vi "DQMH Controls Panel.vi"() -> ()   [LabVIEW 2019, in "Panther Dashboard.lvlib"]
uses:
  Panther Dashboard.lvlib
  Controls/Add.ctl
  Controls/Trash.ctl
  Controls/Convert.ctl
  Controls/rename.ctl
  Controls/Unit Testing.ctl
  Controls/Template.ctl
  Controls/Validate.ctl
  Controls/tester.ctl
  Controls/Antidoc.ctl
  Controls/Info.ctl
  Controls/Theme.ctl
  Controls/Open Document.ctl
  DQMH Tools Menu--enum.ctl
panel:
  in  "Open Documentation":T1 caption="Open\nDocumentation"
  in  "Theme":T2
  in  "About":T3
  in  "Add Event":T4 caption="Add\nEvent"
  in  "Remove Event":T5 caption="Remove\nEvent"
  in  "Convert Event":T6 caption="Convert\nEvent"
  in  "Rename Event":T7 caption="Rename\nEvent"
  in  "Add Module":T4 caption="Add\nModule"
  in  "Rename Module":T7 caption="Rename\nModule"
  in  "Validate Module":T8 caption="Validate\nModule"
  in  "Create Module Template":T9 caption="Create\nTemplate"
  in  "Add Unit Test":T10 caption="Add \nUnit Test"
  in  "Create RT Tester":T11 caption="Create RT\nTester"
  in  "Generate Antidoc":T12 caption="Generate\nAntidoc"
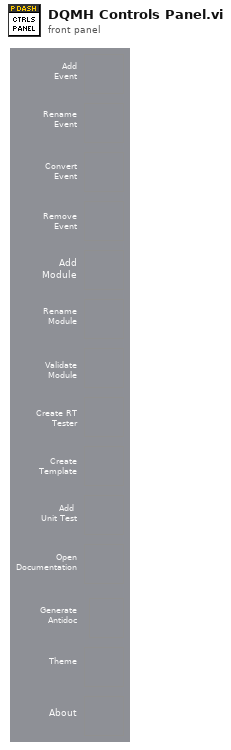
[diagram p1: front panel]
types:
  T1 = typedef "Open Document.ctl" = bool
  T2 = typedef "Theme.ctl" = bool
  T3 = typedef "Info.ctl" = bool
  T4 = typedef "Add.ctl" = bool
  T5 = typedef "Trash.ctl" = bool
  T6 = typedef "Convert.ctl" = bool
  T7 = typedef "rename.ctl" = bool
  T8 = typedef "Validate.ctl" = bool
  T9 = typedef "Template.ctl" = bool
  T10 = typedef "Unit Testing.ctl" = bool
  T11 = typedef "tester.ctl" = bool
  T12 = typedef "Antidoc.ctl" = bool
  T13 = typedef "Panther Dashboard.lvlib/Broadcast Events--cluster.ctl" = cluster{"Module Did Init":refnum<user-event>, "Status Updated":refnum<user-event>, "Error Reported":refnum<user-event>, "Module Did Stop":refnum<user-event>, "Update Module Execution Status":refnum<user-event>, "References Updated":refnum<user-event>, "Projects Updated":refnum<user-event>, "Targets Updated":refnum<user-event>, "Progress updated":refnum<user-event>, "Scale Updated":refnum<user-event>, "Connector Pane Updated":refnum<user-event>, "Documentation Updated":refnum<user-event>, "Module Type Updated":refnum<user-event>}
  T14 = typedef "Panther Dashboard.lvlib/DQMH Tools Menu--enum.ctl" = enum16{"Create New DQMH Event", "Remove DQMH Event", "Convert DQMH Event", "Rename DQMH Event", "Add New DQMH Module", "Create RT Tester", "Rename DQMH Module", "Validate DQMH Module", "Create DQMH Module Template", "New DQMH  Unit Test"}
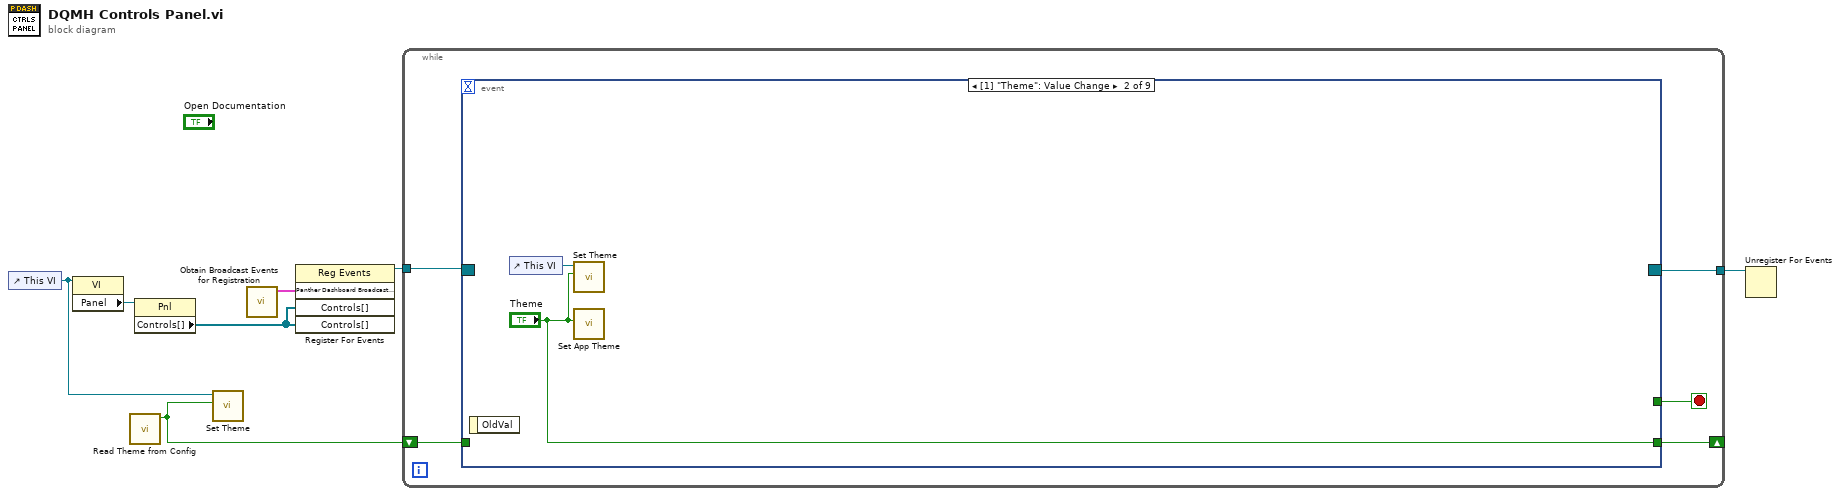
[diagram p0: block diagram]
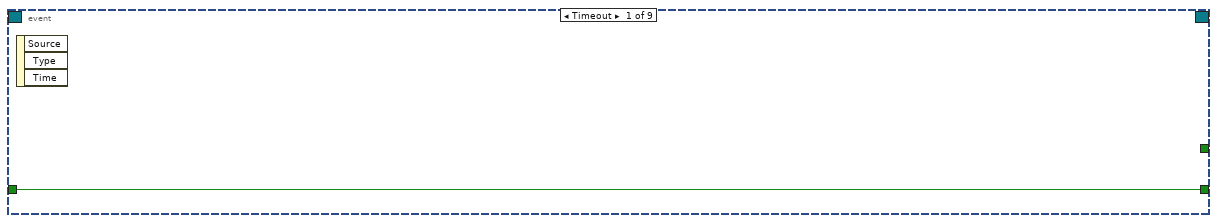
[diagram p2: hidden frame]
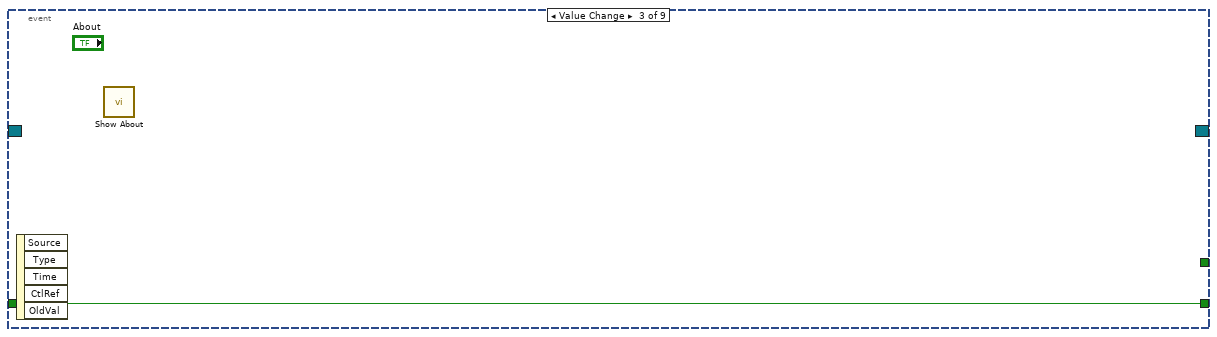
[diagram p3: hidden frame]
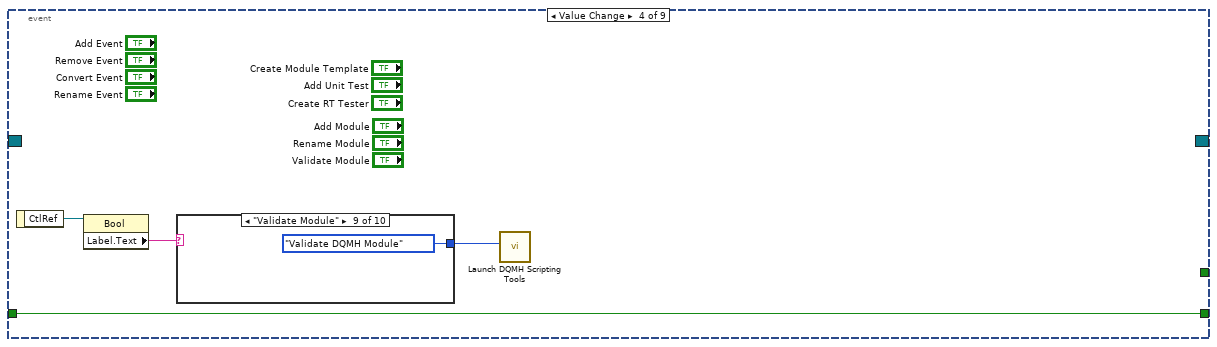
[diagram p4: hidden frame]
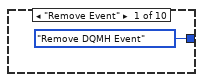
[diagram p5: hidden frame]
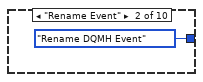
[diagram p6: hidden frame]
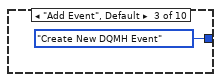
[diagram p7: hidden frame]
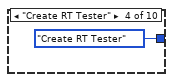
[diagram p8: hidden frame]
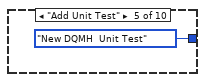
[diagram p9: hidden frame]
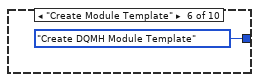
[diagram p10: hidden frame]
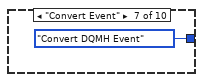
[diagram p11: hidden frame]
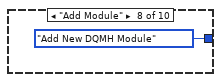
[diagram p12: hidden frame]
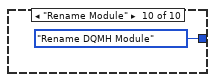
[diagram p13: hidden frame]
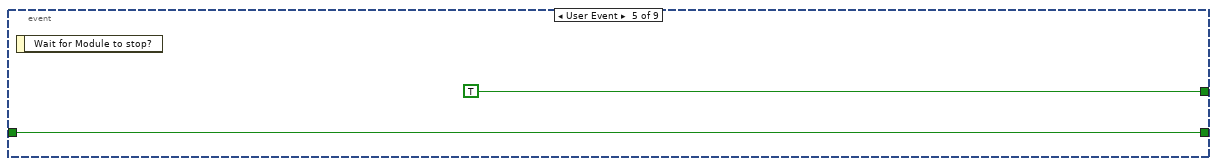
[diagram p14: hidden frame]
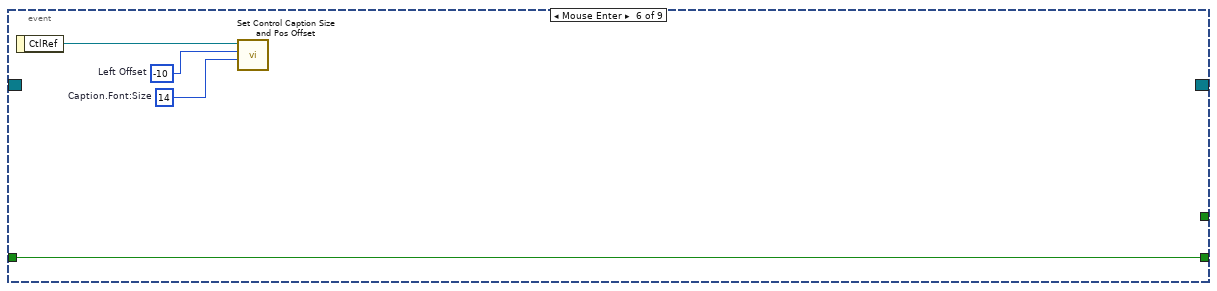
[diagram p15: hidden frame]
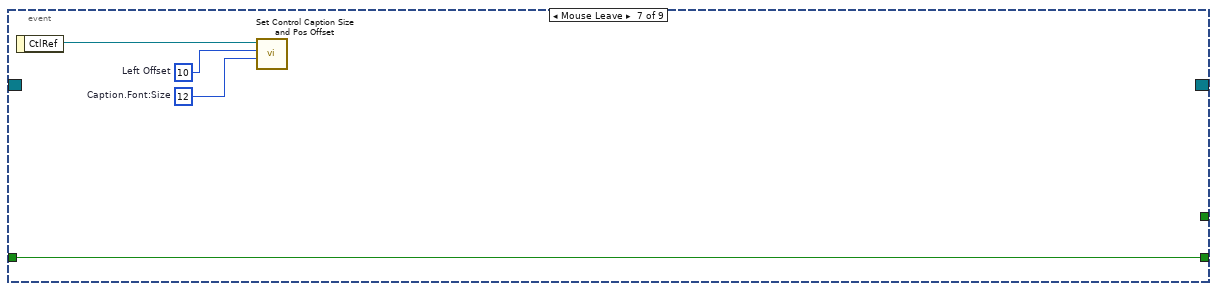
[diagram p16: hidden frame]
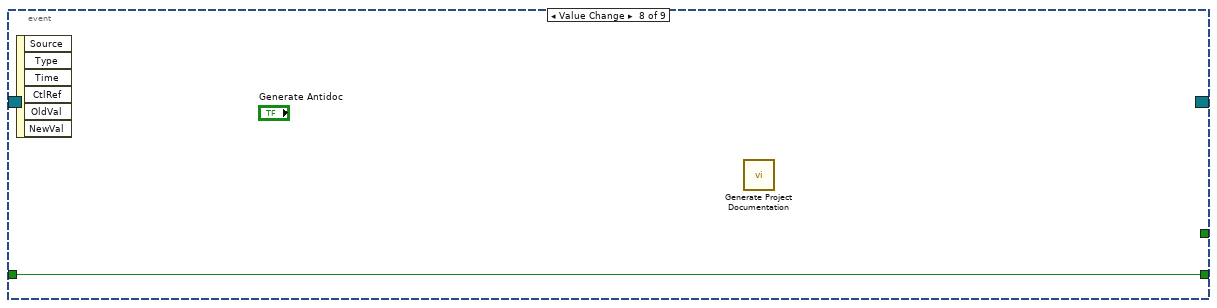
[diagram p17: hidden frame]
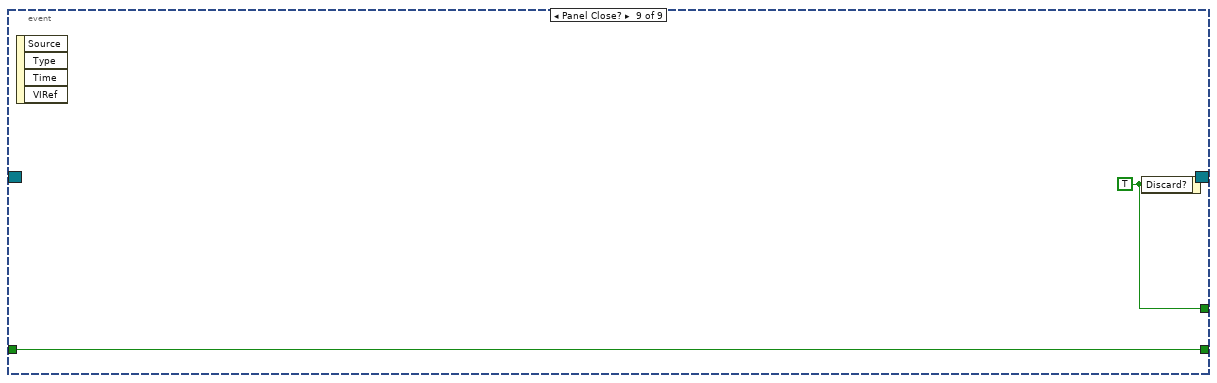
[diagram p18: hidden frame]
diagram:
  n1 = control-ref of="This VI"() -> (w4:refnum<vi>)
  n2 = property class="VI"(reference=w4) -> ("Panel"=w3:refnum<vi>)  [unwired: 1 in, 2 out]
  n3 = call "Read Theme from Config.vi"() -> ("Theme"=w1:bool)  [unwired: 10 in, 1 out]
  n4 = property class="Pnl"(reference=w3) -> ("Controls[]"=w2:refnum<vi>[])  [unwired: 1 in, 2 out]
  n5 = call "Set Theme.vi"("Dark?"=w1, "VI in"=w4) -> ()  [unwired: 10 in]
  n6 = call "Obtain Broadcast Events for Registration.vi"() -> ("Panther Dashboard Broadcast Events"=w6:T13)  [unwired: 9 in, 2 out]
  n7 = register-events(w6, w2, w2) -> (reference out=w7:refnum<event-registration>)  [unwired: 2 in, 1 out]
  n8 = while {
    tunnel: w7 -> [w12]
    tunnel: [w10] -> w5
    shift-right: [w8] -> _
    shift-left: w1 -> [w9]
    stop <- w11 stop-if-true
    n9 = event shown="[1] \"Theme\": Value Change" {
      selector: w12 -> [_ _ _ _ _ _ _ _ _]
      dyn-events: [_ _ _ _ _ _ _ _ _] -> w10
      timeout: _ -> [_ _ _ _ _ _ _ _ _]
      tunnel: [_ _ _ _ TRUE _ _ _ w43] -> w11
      tunnel: w9 -> [w13 _ w16 w17 w31 w36 w40 w41 w42]
      tunnel: [w13 "Theme" w16 w17 w31 w36 w40 w41 w42] -> w8
      event Timeout {
        n10 = event-data() -> ()  [unwired: 1 in, 3 out]
      }
      event Value Change {
        n11 = event-data() -> ()  [unwired: 1 in, 1 out]
        n12 = control-ref of="This VI"() -> (w15:refnum<vi>)
        n13 = call "Set Theme.vi"("Dark?"="Theme", "VI in"=w15) -> ()  [unwired: 10 in]
        n14 = call "Set App Theme.vi"("Theme"="Theme") -> ()  [unwired: 10 in, 1 out]
      }
      event Value Change {
        n15 = event-data() -> ()  [unwired: 1 in, 5 out]
        n16 = call "Show About.vi"() -> ()  [unwired: 11 in, 1 out]
      }
      event Value Change {
        n17 = event-data() -> ("CtlRef"=w20:refnum<vi>)  [unwired: 1 in]
        n18 = property class="Bool"(reference=w20) -> ("Label.Text"=w19:string)  [unwired: 1 in, 2 out]
        n19 = case shown="\"Validate Module\"" w19 {
          tunnel: [DQMH_Tools_Menu--enum."Remove DQMH Event" ("DQMH Tools") DQMH_Tools_Menu--enum."Rename DQMH Event" ("DQMH Tools") DQMH_Tools_Menu--enum."Create New DQMH Event" ("DQMH Tools") DQMH_Tools_Menu--enum."Create RT Tester" ("DQMH Tools") DQMH_Tools_Menu--enum."New DQMH  Unit Test" ("DQMH Tools") DQMH_Tools_Menu--enum."Create DQMH Module Template" ("DQMH Tools") DQMH_Tools_Menu--enum."Convert DQMH Event" ("DQMH Tools") DQMH_Tools_Menu--enum."Add New DQMH Module" ("DQMH Tools") DQMH_Tools_Menu--enum."Validate DQMH Module" ("DQMH Tools") DQMH_Tools_Menu--enum."Rename DQMH Module" ("DQMH Tools")] -> w18
          frame "Remove Event" {
          }
          frame "Rename Event" {
          }
          frame "Add Event", Default {
          }
          frame "Create RT Tester" {
          }
          frame "Add Unit Test" {
          }
          frame "Create Module Template" {
          }
          frame "Convert Event" {
          }
          frame "Add Module" {
          }
          frame "Validate Module" {
          }
          frame "Rename Module" {
          }
        }
        n20 = call "Launch DQMH Scripting Tools.vi"("Scripting Tool"=w18) -> ()  [unwired: 10 in, 1 out]
      }
      event User Event {
        n21 = event-data() -> ()  [unwired: 1 in, 1 out]
      }
      event Mouse Enter {
        w33 = -10  # Left Offset
        w34 = u32 14  # Caption.Font:Size
        n22 = event-data() -> ("CtlRef"=w35:refnum<vi>)  [unwired: 1 in]
        n23 = call "Set Control Caption Size and Pos Offset.vi"("Caption.Font:Size"=w34, "Left Offset"=w33, "Control in"=w35) -> ()  [unwired: 9 in]
      }
      event Mouse Leave {
        w38 = 10  # Left Offset
        w39 = u32 12  # Caption.Font:Size
        n24 = event-data() -> ("CtlRef"=w37:refnum<vi>)  [unwired: 1 in]
        n25 = call "Set Control Caption Size and Pos Offset.vi"("Caption.Font:Size"=w39, "Left Offset"=w38, "Control in"=w37) -> ()  [unwired: 9 in]
      }
      event Value Change {
        n26 = event-data() -> ()  [unwired: 1 in, 6 out]
        n27 = call "Generate Project Documentation.vi"() -> ()  [unwired: 11 in, 1 out]
      }
      event Panel Close? {
        w43 = TRUE ("Discard?")
        n28 = event-data() -> ()  [unwired: 1 in, 4 out]
        n29 = event-data("Discard?"=w43) -> ()  [unwired: 1 in, 1 out]
      }
    }
  }
  n30 = Unregister For Events(event registration refnum=w5) -> ()  [unwired: 1 in, 1 out]
